vi "NB_ReadAttribute.vi"(8 "error in (no error)":errorcluster, 11 "object in":refnum<class "NativeBaseTemplate_4x4x4.lvclass">) -> (0 "error out":errorcluster, 3 "object out":refnum<class "NativeBaseTemplate_4x4x4.lvclass">)   [LabVIEW 2012, in "NativeBaseTemplate_4x4x4.lvclass"]
uses:
  <resource>/Framework/Providers/Open_GDS/ClassProviders/Provider_LvNativeClass/Templates/NativeBaseTemplate_4x4x4/NativeBaseTemplate_4x4x4.lvclass
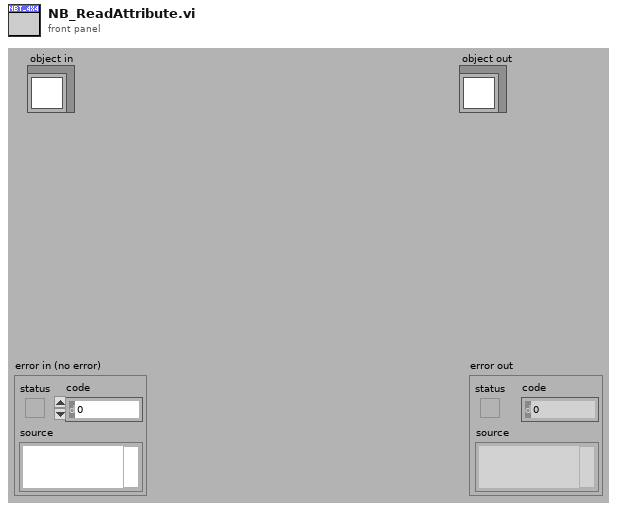
[diagram p1: front panel]
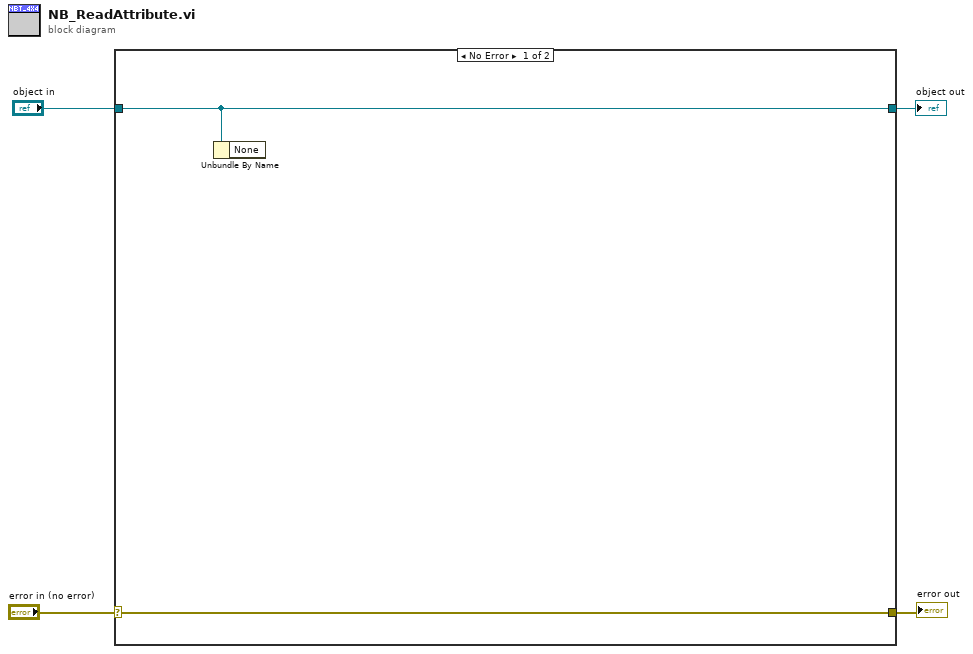
[diagram p0: block diagram]
diagram:
  n1 = case shown="No Error" "error in (no error)" {
    selector: "error in (no error)" -> [w6 w8]
    tunnel: [w6 w8] -> w3
    tunnel: [w5 w7] -> w1
    tunnel: "object in" -> [w5 w7]
    frame No Error {
      n2 = Unbundle By Name(w5) -> ()  [unwired: 1 out]
    }
    frame Error {
    }
  }
  "error out" <- w3
  "object out" <- w1
